vi "Go to Coordinate.vi"(0 "Current Mode":dbl, 1 "Motor Refs":T2[](array[typedef]), 2 "Position":cluster{"X":dbl, "Y":dbl, "Angle":dbl}, 3 "Current Angle (radians; 0 = right)":dbl, 4 "New Command":bool, 5 "Ticks Per Inch":dbl, 6 "Angle Tolerances 1":dbl, 7 "Face angle?":bool, 8 "Angle Tolerances 2":dbl, 9 "Max  Wheel Speed (TPS)":dbl=2100.0, 10 "PID Gains":T1 {"derivative time (Td, min)" format="%.3f"; "integral time (Ti, min)" format="%.3f"; "proportional gain (Kc)" format="%.3f"}, 11 "Speed Setpoint":dbl=0.3) -> (14 "New Mode":dbl, 15 "Left Setpoint":dbl, 16 "Right Setpoint":dbl, 19 "Finished?":bool)   [LabVIEW 2015]
uses:
  <vilib>/Rock Robotics/WPI/MotorControl/WPI_MotorControlDeviceRef.ctl
  <vilib>/Rock Robotics/WPI/MotorControl/WPI_MotorControlType.ctl
  <vilib>/Rock Robotics/SystemInterfaces/DIO/FPGA_DIOPWMChannel.ctl
  <vilib>/Rock Robotics/WPI/PWM/WPI_PWMDeadband.ctl
  <vilib>/Rock Robotics/WPI/CAN/Jaguar/SubVIs/WPI_CANJaguar_ControlMode.ctl
  <vilib>/Rock Robotics/WPI/CAN/TalonSRX/WPI_CANTalonSRX_APIControlMode.ctl
  Support Code/Team900-VIs/Team900SwerveDrive/Team900SwerveDrive.lvlib
panel:
  in  "Distance Tolerances":dbl
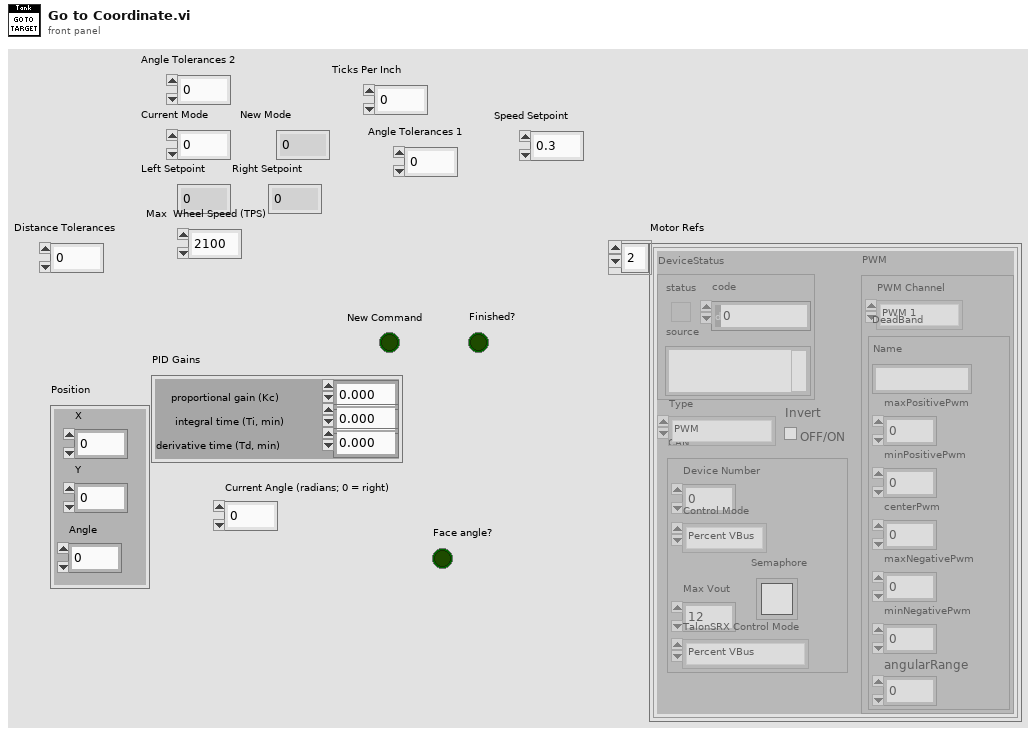
[diagram p1: front panel]
types:
  T1 = cluster{"proportional gain (Kc)":dbl, "integral time (Ti, min)":dbl, "derivative time (Td, min)":dbl}
  T2 = typedef "WPI_MotorControlDeviceRef.ctl" = cluster{"DeviceStatus":errorcluster, "Type":T3, "PWM":cluster{"PWM Channel":T4, "DeadBand":T5}, "CAN":cluster{"Device Number":u8, "Control Mode":T6, "Semaphore":T7, "Max Vout":dbl, "TalonSRX Control Mode":T8}, "Invert":bool}
  T3 = typedef "WPI_MotorControlType.ctl" = enum16{"PWM", "CAN", "CANTalonSRX"}
  T4 = typedef "FPGA_DIOPWMChannel.ctl" = enum8{"PWM 0", "PWM 1", "PWM 2", "PWM 3", "PWM 4", "PWM 5", "PWM 6", "PWM 7", "PWM 8", "PWM 9", "PWM MXP 0", "PWM MXP 1", "PWM MXP 2", "PWM MXP 3", "PWM MXP 4", "PWM MXP 5", "PWM MXP 6", "PWM MXP 7", "PWM MXP 8", "PWM MXP 9", "Invalid"}
  T5 = typedef "WPI_PWMDeadband.ctl" = cluster{"Name":string, "maxPositivePwm":i32, "minPositivePwm":i32, "centerPwm":i32, "maxNegativePwm":i32, "minNegativePwm":i32, "angularRange":u16}
  T6 = typedef "WPI_CANJaguar_ControlMode.ctl" = enum8{"Percent VBus", "Current", "Speed", "Position", "Voltage"}
  T7 = typedef "Semaphore RefNum" = refnum<k1>
  T8 = typedef "WPI_CANTalonSRX_APIControlMode.ctl" = enum8{"Percent VBus", "Speed", "Position", "Slave", "Unchanged / Invalid", "Voltage Compensation", "Current", "Motion Profile"}
  T9 = typedef "WPI_CANTalonSRX_GlobalStatus.ctl" = cluster{"Applied Throttle":dbl, "Module Enabled":bool, "CAN Error":errorcluster, "Closed Loop Error":dbl, "Forward Limit Switch Closed":bool, "Reverse Limit Switch Closed":bool, "Sensor Position":dbl, "Sensor Velocity":dbl, "Current":dbl, "Sticky Fault - Over Temp":bool, "Sticky Fault - Under Voltage":bool, "Sticky Fault - Forward Limit":bool, "Sticky Fault - Reverse Limit":bool, "Sticky Fault - Forward Soft Limit":bool, "Sticky Fault - Reverse Soft Limit":bool, "Brake is Enabled":bool, "Encoder Position":dbl, "Encoder Velocity":dbl, "Encoder Index Count":dbl, "Encoder A Pin State":bool, "Encoder B Pin State":bool, "Encoder Index Pin State":bool, "Analog In":dbl, "Analog In Velocity":dbl, "Temperature (C)":dbl, "Battery Voltage":dbl, "Control 5 Is Supported":bool, "Current Profile Slot Select":dbl, "Pos Div 8":bool, "Vel Div 4":bool, "Pulse Width Position":i32, "Pulse Width Velocity":i32, "Pulse Width Rise To Rise (us)":i32, "Pulse Width Rise To Fall (us)":i32, "Mot Prof Active Is Under Run":bool, "Mot Prof Active Has Under Run":bool, "Mot Prof Active Is Last":bool, "Mot Prof Active Velocity Only":bool, "Mot Prof Active Is Valid":bool, "Mot Prof Buffer Is Full":bool, "Mot Prof Active Profile Slot Select":i32, "Mot Prof NextID":i32, "Mot Prof Count":i32, "Mot Prof Active Velocity":dbl, "Mot Prof Active Position":dbl, "Mot Prof Output Enable":i32}
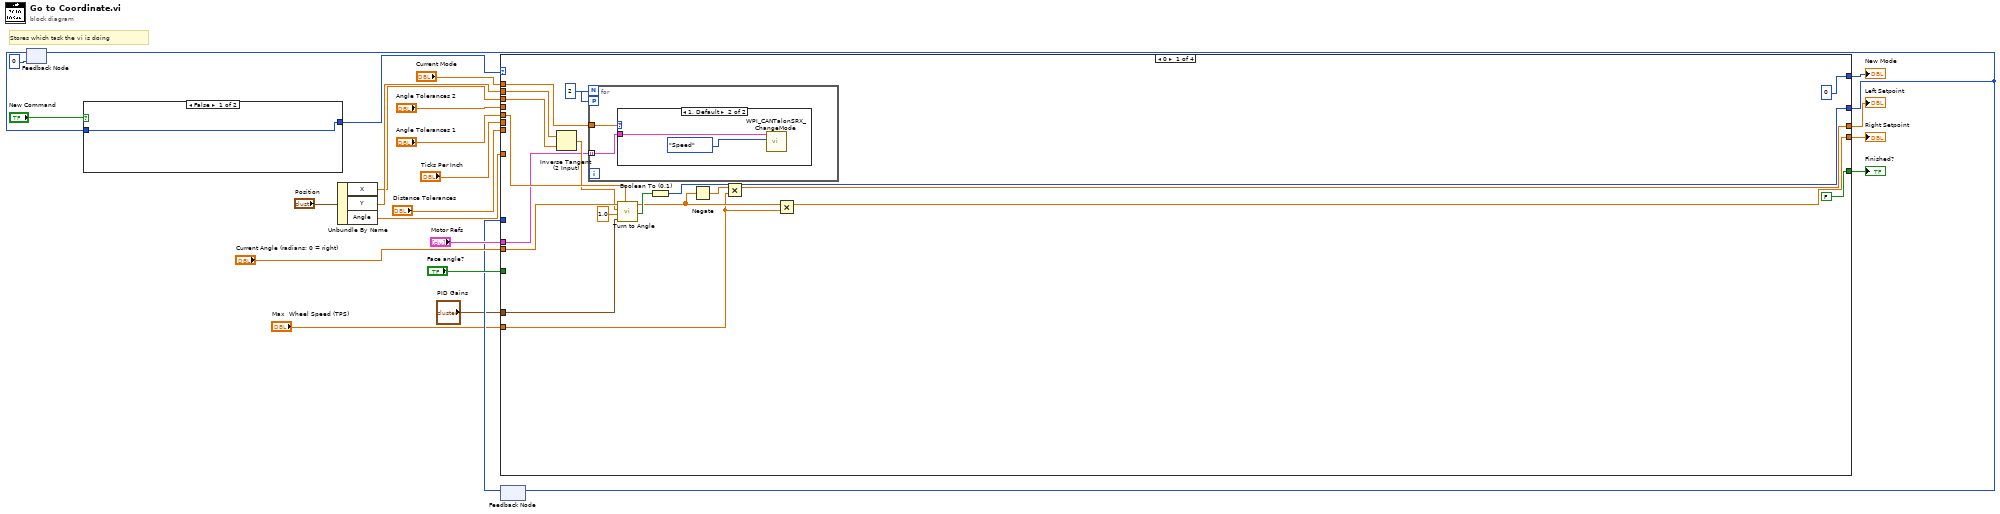
[diagram p0: block diagram]
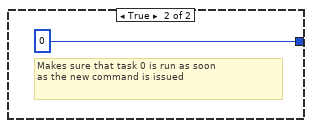
[diagram p2: hidden frame]
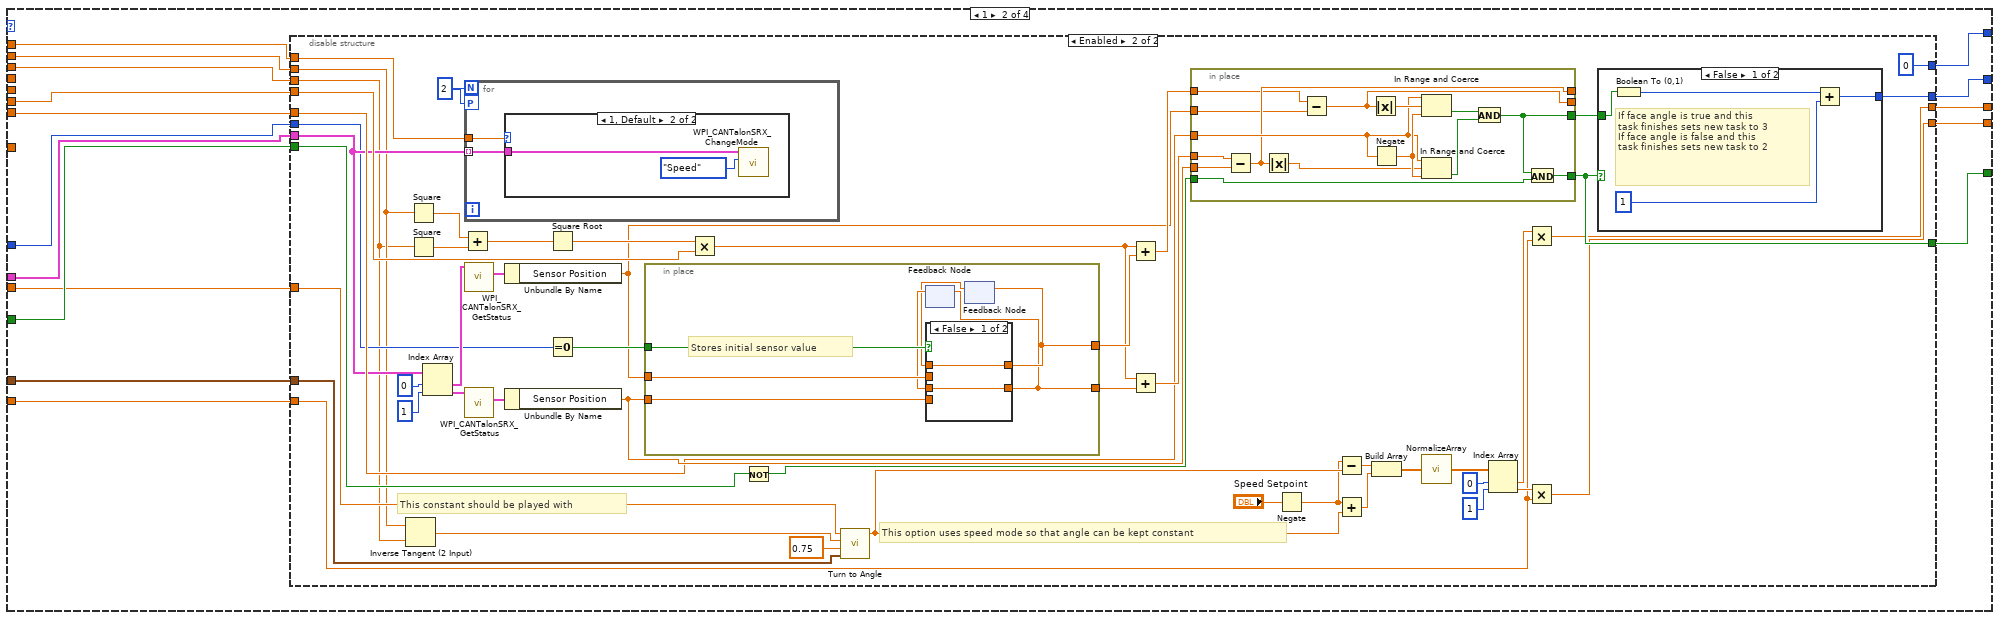
[diagram p4: hidden frame]
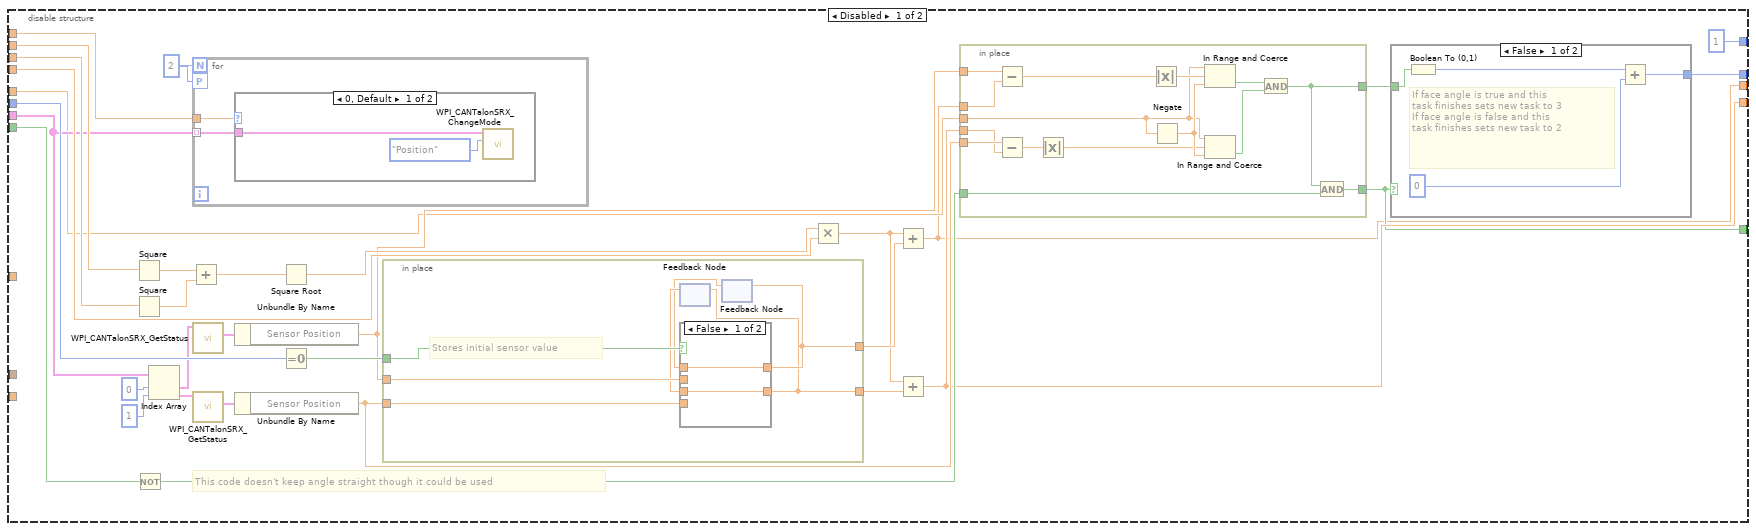
[diagram p5: hidden frame]
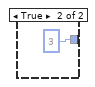
[diagram p6: hidden frame]
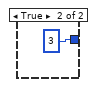
[diagram p9: hidden frame]
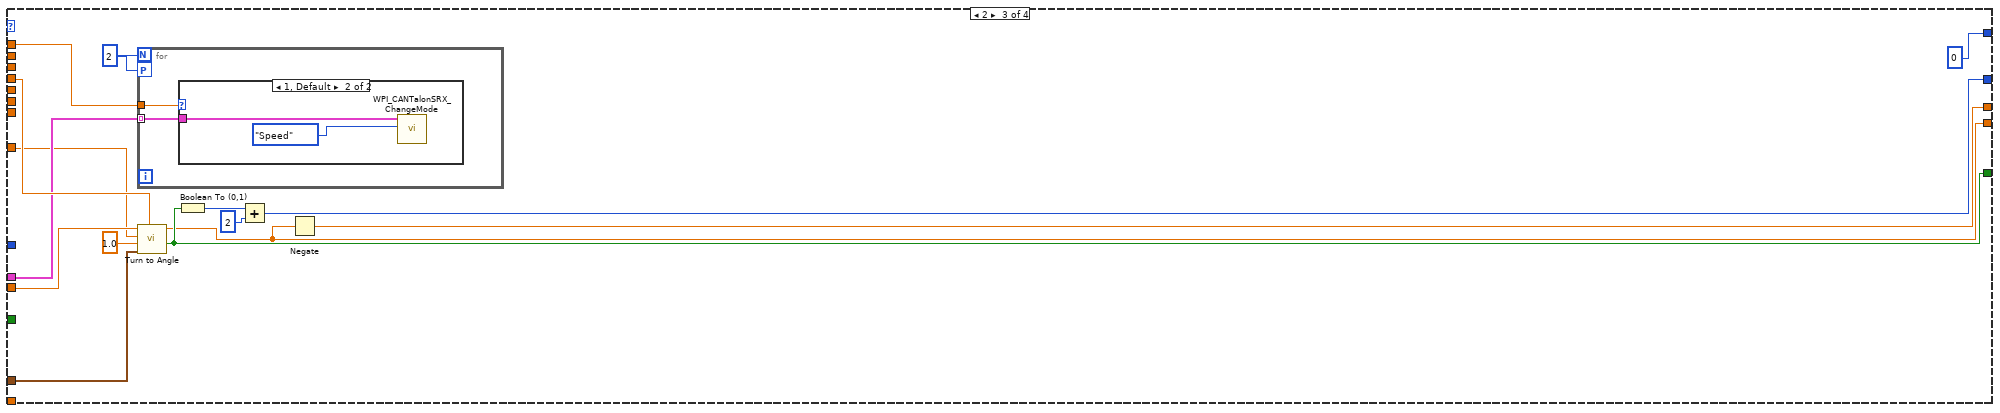
[diagram p12: hidden frame]
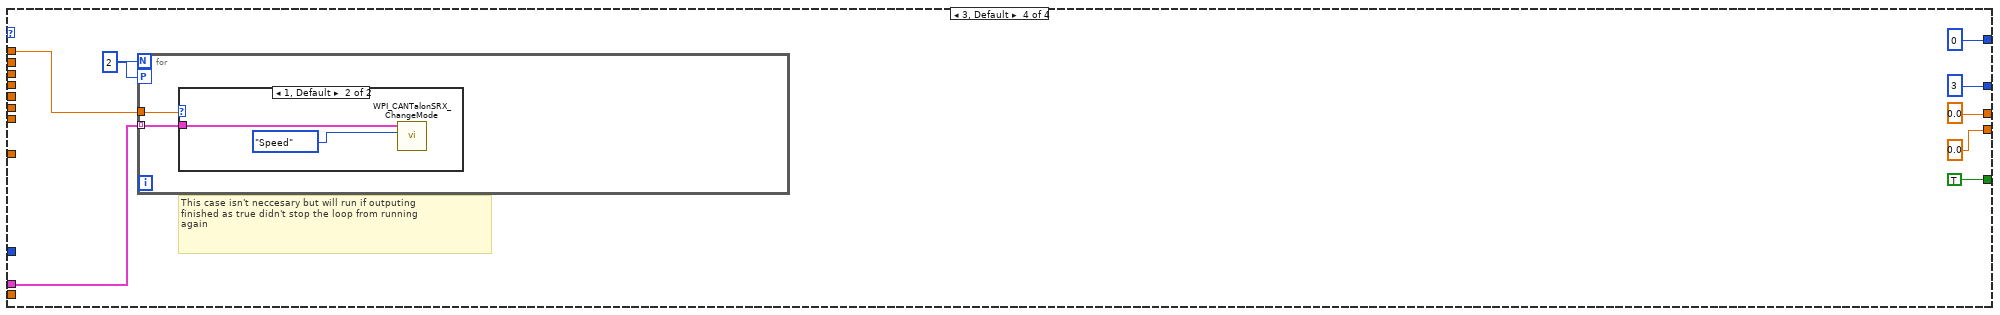
[diagram p14: hidden frame]
diagram:
  # "Stores which task the vi is doing"
  n1 = feedback #1(0) -> (w5:i32)
  n2 = case shown="False" "New Command" {
    tunnel: [w25 0] -> w6
    tunnel: w5 -> [w25 _]
    frame False {
    }
    frame True {
      # "Makes sure that task 0 is run as soon \nas the new command is issued"
    }
  }
  n3 = Unbundle By Name("Position") -> ("X"=w10:dbl, "Y"=w22:dbl, "Angle"=w12:dbl)
  n4 = feedback #2() -> (w8:i32)  [unwired: 1 in]
  n5 = case shown="0" w6 {
    tunnel: "Current Angle (radians; 0 = right)" -> [w45 w53 w222 _]
    tunnel: "Angle Tolerances 1" -> [w44 _ _ _]
    tunnel: w22 -> [w43 w65 _ _]
    tunnel: w10 -> [w42 w64 _ _]
    tunnel: [w32 w54 w230 3] -> w4
    tunnel: "Angle Tolerances 2" -> [_ _ w229 _]
    tunnel: [FALSE w55 w228 TRUE] -> w20
    tunnel: "Motor Refs" -> [w38 w58 w227 w239]
    tunnel: "Current Mode" -> [w37 w61 w226 w238]
    tunnel: [0 w63 0 0] -> w18
    tunnel: [w29 w52 w224 0.0] -> w17
    tunnel: [w28 w57 w223 0.0] -> w16
    tunnel: "Ticks Per Inch" -> [_ w62 _ _]
    tunnel: "Face angle?" -> [_ w60 _ _]
    tunnel: w12 -> [_ _ w220 _]
    tunnel: w8 -> [_ w59 _ _]
    tunnel: "Distance Tolerances" -> [_ w56 _ _]
    tunnel: "Max  Wheel Speed (TPS)" -> [w27 w51 _ _]
    tunnel: "PID Gains" -> [w30 w50 w218 _]
    frame 0 {
      w33 = 2
      n6 = Inverse Tangent (2 Input)(1:w42, 2:w43) -> (0:w41:dbl)
      n7 = for {
        N: w33 -> [_]
        tunnel: w38 -> [w47] mode=indexing
        tunnel: w37 -> [w46]
        workers-P: w33 -> [_]
        n8 = case shown="1, Default" w46 {
          tunnel: w47 -> [_ w49]
          frame 0 {
          }
          frame 1, Default {
            n9 = call <vilib>:"WPI_CANTalonSRX_ChangeMode.vi"("Control Mode"=WPI_CANTalonSRX_APIControlMode."Speed", "CAN Talon SRX Ref"=w49) -> ()  [unwired: 8 in, 2 out]
          }
        }
      }
      n10 = call "Turn to Angle.vi"("Angle Tolerance"=w44, "PID Gains"=w30, "Rotation Multiplier"=1.0, "Target angle"=w41, "Angle (radians; 0 = right)"=w45) -> ("Finished?"=w40:bool, "Turn Set Point"=w34:dbl)  [unwired: 2 in]
      n11 = Boolean To (0,1)(Boolean=w40) -> (0, 1=w32:i16)
      n12 = Negate(x=w34) -> (-x=w35:dbl)
      n13 = Multiply(x=w35, y=w27) -> (x*y=w29:dbl)
      n14 = Multiply(x=w34, y=w27) -> (x*y=w28:dbl)
    }
    frame 1 {
      n15 = disable-structure shown="Enabled" {
        disable-tunnel: w65 -> [w97 w151]
        disable-tunnel: w64 -> [w96 w150]
        disable-tunnel: [1 0] -> w63
        disable-tunnel: w62 -> [w90 w158]
        disable-tunnel: w61 -> [w89 w160]
        disable-tunnel: w60 -> [w87 w155]
        disable-tunnel: w59 -> [w85 w156]
        disable-tunnel: w58 -> [w83 w157]
        disable-tunnel: [w72 w146] -> w57
        disable-tunnel: w56 -> [w70 w159]
        disable-tunnel: [w69 w162] -> w55
        disable-tunnel: [w68 w163] -> w54
        disable-tunnel: w53 -> [_ w152]
        disable-tunnel: w51 -> [_ w136]
        disable-tunnel: [w66 w145] -> w52
        disable-tunnel: w50 -> [_ w135]
        frame Disabled {
          w88 = 2
          # "This code doesn't keep angle straight though it could be used"
          n16 = Square(x=w97) -> (x^2=w94:dbl)
          n17 = Square(x=w96) -> (x^2=w95:dbl)
          n18 = Not(x=w87) -> (.not. x?=w86:bool)
          n19 = Index Array(array=w83, index #1=0 ("index"), index #2=1 ("index")) -> (element #1=w80:T2, element #2=w78:T2)
          n20 = Add(x=w94, y=w95) -> (x+y=w93:dbl)
          n21 = for {
            N: w88 -> [_]
            tunnel: w83 -> [w130] mode=indexing
            tunnel: w89 -> [w129]
            workers-P: w88 -> [_]
            n22 = case shown="0, Default" w129 {
              tunnel: w130 -> [w132 _]
              frame 0, Default {
                n23 = call <vilib>:"WPI_CANTalonSRX_ChangeMode.vi"("Control Mode"=WPI_CANTalonSRX_APIControlMode."Position", "CAN Talon SRX Ref"=w132) -> ()  [unwired: 8 in, 2 out]
              }
              frame 1 {
              }
            }
          }
          n24 = call <vilib>:"WPI_CANTalonSRX_GetStatus.vi"("CAN Talon SRX Ref"=w80) -> ("Talon SRX Status"=w79:T9)  [unwired: 8 in, 2 out]
          n25 = call <vilib>:"WPI_CANTalonSRX_GetStatus.vi"("CAN Talon SRX Ref"=w78) -> ("Talon SRX Status"=w77:T9)  [unwired: 8 in, 2 out]
          n26 = Unbundle By Name(w79) -> ("Sensor Position"=w71:dbl)
          n27 = Unbundle By Name(w77) -> ("Sensor Position"=w73:dbl)
          n28 = Square Root(x=w93) -> (sqrt(x)=w91:dbl)
          n29 = Equal To 0?(x=w85) -> (x = 0?=w84:bool)
          n30 = in-place {
            in-place-border: w84 -> [w124]
            in-place-border: w71 -> [w123]
            in-place-border: w73 -> [w122]
            in-place-border: [w121] -> w76
            in-place-border: [w118] -> w74
            # "Stores initial sensor value"
            n31 = feedback #3() -> (w120:dbl)  [unwired: 1 in]
            n32 = feedback #4() -> (w119:dbl)  [unwired: 1 in]
            n33 = case shown="False" w124 {
              tunnel: [w126 w128] -> w121
              tunnel: w123 -> [_ w128]
              tunnel: w119 -> [w126 _]
              tunnel: [w125 w127] -> w118
              tunnel: w122 -> [_ w127]
              tunnel: w120 -> [w125 _]
              frame False {
              }
              frame True {
              }
            }
            n34 = feedback-in #3(w118) -> ()
            n35 = feedback-in #4(w121) -> ()
          }
          n36 = Multiply(x=w91, y=w90) -> (x*y=w75:dbl)
          n37 = Add(x=w75, y=w76) -> (x+y=w66:dbl)
          n38 = Add(x=w75, y=w74) -> (x+y=w72:dbl)
          n39 = in-place {
            in-place-border: w86 -> [w112]
            in-place-border: w73 -> [w111]
            in-place-border: w72 -> [w110]
            in-place-border: w71 -> [w108]
            in-place-border: w66 -> [w107]
            in-place-border: w70 -> [w98]
            in-place-border: [w100] -> w69
            in-place-border: [w99] -> w67
            n40 = Subtract(x=w108, y=w107) -> (x-y=w106:dbl)
            n41 = Subtract(x=w111, y=w110) -> (x-y=w109:dbl)
            n42 = Absolute Value(x=w109) -> (abs(x)=w103:dbl)
            n43 = Absolute Value(x=w106) -> (abs(x)=w104:dbl)
            n44 = Negate(x=w98) -> (-x=w105:dbl)
            n45 = In Range and Coerce(upper limit=w98, x=w104, lower limit=w105) -> (In Range?=w102:bool)  [unwired: 1 out]
            n46 = In Range and Coerce(upper limit=w98, x=w103, lower limit=w105) -> (In Range?=w101:bool)  [unwired: 1 out]
            n47 = And(x=w102, y=w101) -> (x .and. y?=w99:bool)
            n48 = And(x=w99, y=w112) -> (x .and. y?=w100:bool)
          }
          n49 = case shown="False" w69 {
            tunnel: [w113 3] -> w68
            tunnel: w67 -> [w116 _]
            frame False {
              # "If face angle is true and this \ntask finishes sets new task to 3\nIf face angle is false and this \ntask finishes sets new task to 2"
              n50 = Boolean To (0,1)(Boolean=w116) -> (0, 1=w115:i16)
              n51 = Add(x=w115, y=0) -> (x+y=w113:i32)
            }
            frame True {
            }
          }
        }
        frame Enabled {
          w178 = 2
          # "This constant should be played with"
          # "This option uses speed mode so that angle can be kept constant"
          n52 = Inverse Tangent (2 Input)(1:w150, 2:w151) -> (0:w149:dbl)
          n53 = Square(x=w151) -> (x^2=w181:dbl)
          n54 = Square(x=w150) -> (x^2=w182:dbl)
          n55 = Index Array(array=w157, index #1=0 ("index"), index #2=1 ("index")) -> (element #1=w173:T2, element #2=w171:T2)
          n56 = Add(x=w181, y=w182) -> (x+y=w180:dbl)
          n57 = for {
            N: w178 -> [_]
            tunnel: w157 -> [w215] mode=indexing
            tunnel: w160 -> [w214]
            workers-P: w178 -> [_]
            n58 = case shown="1, Default" w214 {
              tunnel: w215 -> [_ w217]
              frame 0 {
              }
              frame 1, Default {
                n59 = call <vilib>:"WPI_CANTalonSRX_ChangeMode.vi"("Control Mode"=WPI_CANTalonSRX_APIControlMode."Speed", "CAN Talon SRX Ref"=w217) -> ()  [unwired: 8 in, 2 out]
              }
            }
          }
          n60 = call <vilib>:"WPI_CANTalonSRX_GetStatus.vi"("CAN Talon SRX Ref"=w173) -> ("Talon SRX Status"=w172:T9)  [unwired: 8 in, 2 out]
          n61 = call <vilib>:"WPI_CANTalonSRX_GetStatus.vi"("CAN Talon SRX Ref"=w171) -> ("Talon SRX Status"=w170:T9)  [unwired: 8 in, 2 out]
          n62 = Unbundle By Name(w172) -> ("Sensor Position"=w153:dbl)
          n63 = Unbundle By Name(w170) -> ("Sensor Position"=w166:dbl)
          n64 = Square Root(x=w180) -> (sqrt(x)=w179:dbl)
          n65 = Equal To 0?(x=w156) -> (x = 0?=w176:bool)
          n66 = in-place {
            in-place-border: w176 -> [w209]
            in-place-border: w153 -> [w208]
            in-place-border: w166 -> [w207]
            in-place-border: [w206] -> w169
            in-place-border: [w203] -> w167
            # "Stores initial sensor value"
            n67 = feedback #5() -> (w205:dbl)  [unwired: 1 in]
            n68 = feedback #6() -> (w204:dbl)  [unwired: 1 in]
            n69 = case shown="False" w209 {
              tunnel: [w211 w213] -> w206
              tunnel: w208 -> [_ w213]
              tunnel: w204 -> [w211 _]
              tunnel: [w210 w212] -> w203
              tunnel: w207 -> [_ w212]
              tunnel: w205 -> [w210 _]
              frame False {
              }
              frame True {
              }
            }
            n70 = feedback-in #5(w203) -> ()
            n71 = feedback-in #6(w206) -> ()
          }
          n72 = Multiply(x=w179, y=w158) -> (x*y=w168:dbl)
          n73 = Not(x=w155) -> (.not. x?=w177:bool)
          n74 = call "Turn to Angle.vi"("PID Gains"=w135, "Rotation Multiplier"=0.75, "Target angle"=w149, "Angle (radians; 0 = right)"=w152) -> ("Turn Set Point"=w148:dbl)  [unwired: 3 in, 1 out]
          n75 = Add(x=w168, y=w169) -> (x+y=w154:dbl)
          n76 = Add(x=w168, y=w167) -> (x+y=w161:dbl)
          n77 = in-place {
            in-place-border: w177 -> [w197]
            in-place-border: w166 -> [w186]
            in-place-border: w161 -> [w185]
            in-place-border: w153 -> [w184]
            in-place-border: w154 -> [w183]
            in-place-border: w159 -> [w189]
            in-place-border: [w191] -> w162
            in-place-border: [w190] -> w165
            in-place-border: [w188] -> _
            in-place-border: [w187] -> _
            n78 = Subtract(x=w185, y=w186) -> (x-y=w187:dbl)
            n79 = Absolute Value(x=w187) -> (abs(x)=w194:dbl)
            n80 = Subtract(x=w183, y=w184) -> (x-y=w188:dbl)
            n81 = Absolute Value(x=w188) -> (abs(x)=w195:dbl)
            n82 = Negate(x=w189) -> (-x=w196:dbl)
            n83 = In Range and Coerce(upper limit=w189, x=w195, lower limit=w196) -> (In Range?=w193:bool)  [unwired: 1 out]
            n84 = In Range and Coerce(upper limit=w189, x=w194, lower limit=w196) -> (In Range?=w192:bool)  [unwired: 1 out]
            n85 = And(x=w193, y=w192) -> (x .and. y?=w190:bool)
            n86 = And(x=w190, y=w197) -> (x .and. y?=w191:bool)
          }
          n87 = Negate(x="Speed Setpoint") -> (-x=w133:dbl)
          n88 = Subtract(x=w133, y=w148) -> (x-y=w144:dbl)
          n89 = Add(x=w133, y=w148) -> (x+y=w143:dbl)
          n90 = Build Array(w144, w143) -> (w142:dbl[])
          n91 = call "NormalizeArray.vi"("array"=w142) -> ("normalized array"=w141:dbl[])
          n92 = Index Array(array=w141, index #1=0, index #2=1 ("index")) -> (element #1=w138:dbl, element #2=w137:dbl)
          n93 = Multiply(x=w138, y=w136) -> (x*y=w145:dbl)
          n94 = Multiply(x=w137, y=w136) -> (x*y=w146:dbl)
          n95 = case shown="False" w162 {
            tunnel: [w198 3] -> w163
            tunnel: w165 -> [w201 _]
            frame False {
              # "If face angle is true and this \ntask finishes sets new task to 3\nIf face angle is false and this \ntask finishes sets new task to 2"
              n96 = Boolean To (0,1)(Boolean=w201) -> (0, 1=w200:i16)
              n97 = Add(x=w200, y=1) -> (x+y=w198:i32)
            }
            frame True {
            }
          }
        }
      }
    }
    frame 2 {
      w221 = 2
      n98 = for {
        N: w221 -> [_]
        tunnel: w227 -> [w234] mode=indexing
        tunnel: w226 -> [w233]
        workers-P: w221 -> [_]
        n99 = case shown="1, Default" w233 {
          tunnel: w234 -> [_ w236]
          frame 0 {
          }
          frame 1, Default {
            n100 = call <vilib>:"WPI_CANTalonSRX_ChangeMode.vi"("Control Mode"=WPI_CANTalonSRX_APIControlMode."Speed", "CAN Talon SRX Ref"=w236) -> ()  [unwired: 8 in, 2 out]
          }
        }
      }
      n101 = call "Turn to Angle.vi"("Angle Tolerance"=w229, "PID Gains"=w218, "Rotation Multiplier"=1.0, "Target angle"=w220, "Angle (radians; 0 = right)"=w222) -> ("Finished?"=w228:bool, "Turn Set Point"=w223:dbl)  [unwired: 2 in]
      n102 = Boolean To (0,1)(Boolean=w228) -> (0, 1=w231:i16)
      n103 = Add(x=w231, y=2) -> (x+y=w230:i32)
      n104 = Negate(x=w223) -> (-x=w224:dbl)
    }
    frame 3, Default {
      w240 = 2
      # "This case isn't neccesary but will run if outputing\nfinished as true didn't stop the loop from running\nagain"
      n105 = for {
        N: w240 -> [_]
        tunnel: w239 -> [w246] mode=indexing
        tunnel: w238 -> [w245]
        workers-P: w240 -> [_]
        n106 = case shown="1, Default" w245 {
          tunnel: w246 -> [_ w248]
          frame 0 {
          }
          frame 1, Default {
            n107 = call <vilib>:"WPI_CANTalonSRX_ChangeMode.vi"("Control Mode"=WPI_CANTalonSRX_APIControlMode."Speed", "CAN Talon SRX Ref"=w248) -> ()  [unwired: 8 in, 2 out]
          }
        }
      }
    }
  }
  "Finished?" <- w20
  "New Mode" <- w18
  "Left Setpoint" <- w17
  "Right Setpoint" <- w16
  n108 = feedback-in #1(w4) -> ()
  n109 = feedback-in #2(w4) -> ()
